vi "main.vi"() -> ()   [LabVIEW 2021]
panel:
  in  "Stop":bool
  out "Array 2":i32[](array[numeric])
  in  "y":i32
  out "Array":i32[](array[numeric])
  out "Greeting":string
  in  "String":string
  out "Numeric 3":dbl format="%#.2g"
  in  "Numeric 2":dbl
  in  "Numeric":i32
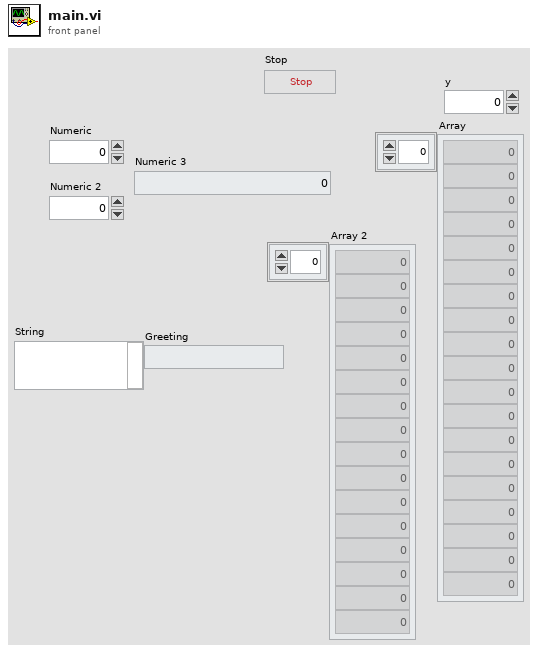
[diagram p1: front panel]
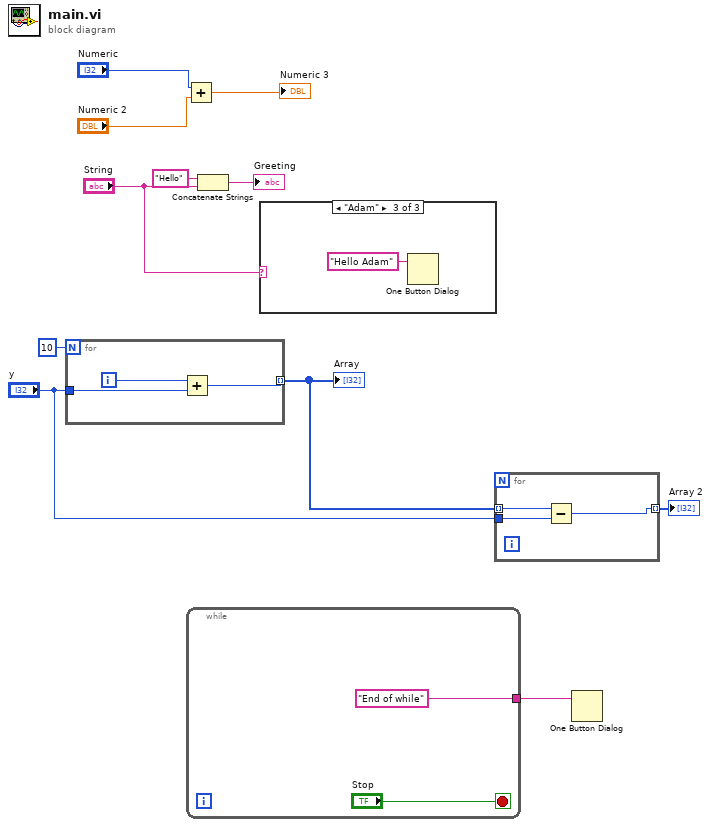
[diagram p0: block diagram]
diagram:
  n1 = for {
    N: 10 -> [_]
    tunnel: [w13] -> w4 mode=indexing
    tunnel: "y" -> [w12]
    i -> [w14]
    n2 = Add(x=w14, y=w12) -> (x+y=w13:i32)
  }
  "Array" <- w4
  n3 = Add(x="Numeric", y="Numeric 2") -> (x+y=→"Numeric 3":dbl)
  n4 = while {
    tunnel: ["End of while"] -> w1
    stop <- "Stop" stop-if-true
  }
  n5 = Concatenate Strings("Hello" ("string"), "String") -> (→"Greeting":string)
  n6 = case shown="\"Adam\"" "String" {
    frame "False", Default {
    }
    frame "Daria" {
    }
    frame "Adam" {
      n7 = One Button Dialog(message="Hello Adam") -> ()  [unwired: 1 in, 1 out]
    }
  }
  n8 = for {
    tunnel: w4 -> [w20] mode=indexing
    tunnel: [w18] -> w3 mode=indexing
    tunnel: "y" -> [w19]
    n9 = Subtract(x=w20, y=w19) -> (x-y=w18:i32)
  }
  "Array 2" <- w3
  n10 = One Button Dialog(message=w1) -> ()  [unwired: 1 in, 1 out]
